vi "CRYUnflatten SoundCard.vi"(11 "Flatten SoundCard":string) -> (0 "Error?":bool=TRUE, 2 "SoundCard":T1={"Name"="", "Analog I/O"=0, "Digital I/O"=0, "Channels"=2, "Dig Dev ID"=1, "N ports"=3, "Interface"=0, "Dig I/O Ports"=[{"port #"=1, "width"=8, "direction"=0}, {"port #"=2, "width"=8, "direction"=0}, {"port #"=3, "width"=8, "direction"=0}], "Interf settings"=[], "N interfs"=3, "udev SNs"=[], "udev enable"=FALSE, "Channel Array"=[], "Cal sequence"="", "SelectedIn"=0, "SelectedOut"=0, "SelectedTab"=0, "State"=FALSE, "Help"="", "Advanced"=FALSE, "In Audio Driver"=0, "Out Audio Driver"=0} {"Channel Array"."Coupling" items=["Default"=-1, "RSE"=10083, "NRSE"=10078, "Differential"=10106, "Pseudodifferential"=12529]; "Channel Array"."term config" items=["Default"=-1, "RSE"=10083, "NRSE"=10078, "Differential"=10106, "Pseudodifferential"=12529]; "Channel Array"."Anti-aliasing Factor (%fs)" format="%.2f"}, 3 "Header info":T3={"Data type"="Data            ", "Version"=1, "Dimensions"=0})   [LabVIEW 2013]
uses:
  Typedef Control/CRYHardware.ctl
  Typedef Control/CRYHardware Channel Info.ctl
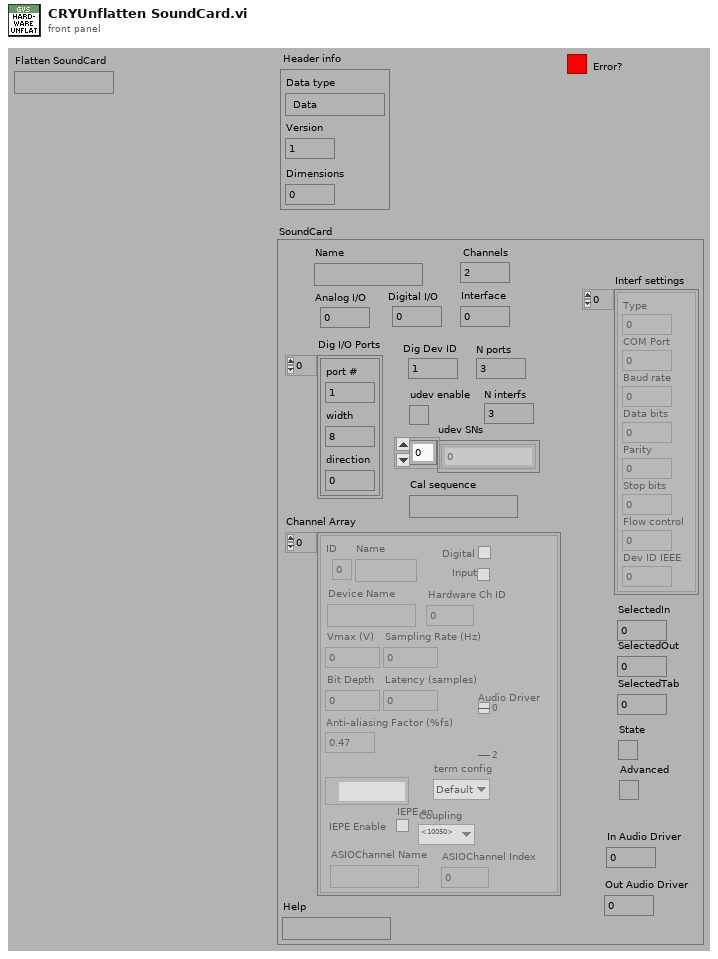
[diagram p1: front panel]
types:
  T1 = typedef "CRYHardware.ctl" = cluster{"Name":string, "Analog I/O":u16, "Digital I/O":u16, "Channels":u8, "Dig Dev ID":u8, "N ports":u8, "Interface":u32, "Dig I/O Ports":cluster{"port #":i16, "width":i16, "direction":i32}[], "Interf settings":cluster{"Type":u16, "COM Port":u8, "Baud rate":u32, "Data bits":u32, "Parity":u16, "Stop bits":u16, "Flow control":u16, "Dev ID IEEE":u8}[], "N interfs":i32, "udev SNs":i16[], "udev enable":bool, "Channel Array":T2[], "Cal sequence":string, "SelectedIn":u16, "SelectedOut":u16, "SelectedTab":u16, "State":bool, "Help":string, "Advanced":bool, "In Audio Driver":u16, "Out Audio Driver":u16}
  T2 = typedef "CRYHardware Channel Info.ctl" = cluster{"ID":i32, "Name":string, "Digital":bool, "Input":bool, "Device Name":string, "Hardware Ch ID":u8, "Vmax (V)":dbl, "Latency (samples)":dbl, "Sampling Rate (Hz)":u32, "Bit Depth":u32, "Anti-aliasing Factor (%fs)":sgl, "DAQmx Channel":tag, "term config":i32, "Coupling":i32, "IEPE en":bool, "ASIOChannel Name":string, "Audio Driver":u16, "ASIOChannel Index":u8}
  T3 = cluster{"Data type":string, "Version":u16, "Dimensions":u8}
  T4 = cluster{"Name":string, "Analog I/O":u16, "Digital I/O":u16, "Channels":u8, "Dig Dev ID":u8, "N ports":u8, "Interface":u32, "Dig I/O Ports":cluster{"port #":i16, "width":i16, "direction":i32}[], "Interf settings":cluster{"Type":u16, "COM Port":u8, "Baud rate":u32, "Data bits":u32, "Parity":u16, "Stop bits":u16, "Flow control":u16, "Dev ID IEEE":u8}[], "N interfs":i32, "udev SNs":i16[], "udev enable":bool, "Channel Array":cluster{"ID":i32, "Name":string, "Digital":bool, "Input":bool, "Device Name":string, "Hardware Ch ID":u8, "Vmax (V)":dbl, "Latency (samples)":dbl, "Sampling Rate (Hz)":u32, "Bit Depth":u32, "Anti-aliasing Factor (%fs)":sgl, "DAQmx Channel":tag, "term config":i32, "Coupling":i32, "IEPE en":bool, "Audio Driver":u16}[], "Cal sequence":string, "SelectedIn":u16, "SelectedOut":u16, "SelectedTab":u16, "State":bool, "Help":string, "Advanced":bool}
  T5 = cluster{"Name":string, "Analog I/O":u16, "Digital I/O":u16, "Channels":u8, "Dig Dev ID":u8, "N ports":u8, "Interface":u32, "Dig I/O Ports":cluster{"port #":i16, "width":i16, "direction":i32}[], "Interf settings":cluster{"Type":u16, "COM Port":u8, "Baud rate":u32, "Data bits":u32, "Parity":u16, "Stop bits":u16, "Flow control":u16, "Dev ID IEEE":u8}[], "N interfs":i32, "udev SNs":i16[], "udev enable":bool, "Channel Array":cluster{"ID":i32, "Name":string, "Digital":bool, "Input":bool, "Device Name":string, "Hardware Ch ID":u8, "Vmax (V)":dbl, "Latency (samples)":dbl, "Sampling Rate (Hz)":u32, "Bit Depth":u32, "Anti-aliasing Factor (%fs)":sgl, "DAQmx Channel":tag, "term config":i32, "Coupling":i32, "IEPE en":bool, "Audio Driver":u16}[], "Cal sequence":string, "SelectedIn":u16, "SelectedOut":u16, "SelectedTab":u16, "State":bool, "Help":string}
  T6 = cluster{"Name":string, "Analog I/O":u16, "Digital I/O":u16, "Channels":u8, "Dig Dev ID":u8, "N ports":u8, "Interface":u32, "Dig I/O Ports":cluster{"port #":i16, "width":i16, "direction":i32}[], "Interf settings":cluster{"Type":u16, "COM Port":u8, "Baud rate":u32, "Data bits":u32, "Parity":u16, "Stop bits":u16, "Flow control":u16, "Dev ID IEEE":u8}[], "N interfs":i32, "udev SNs":i16[], "udev enable":bool, "Channel Array":cluster{"ID":i32, "Name":string, "Digital":bool, "Input":bool, "Device Name":string, "Hardware Ch ID":u8, "Vmax (V)":dbl, "Latency (samples)":dbl, "Sampling Rate (Hz)":u32, "Bit Depth":u32, "Anti-aliasing Factor (%fs)":sgl, "DAQmx Channel":tag, "term config":i32, "Coupling":i32, "IEPE en":bool, "Audio Driver":u16}[], "Cal sequence":string, "SelectedIn":u16, "SelectedOut":u16, "SelectedTab":u16, "State":bool}
  T7 = cluster{"unsigned byte array[0]":u8, "unsigned byte array[1]":u8, "unsigned byte array[2]":u8}
  T8 = cluster{"port #":i16, "width":i16, "direction":i32}[]
  T9 = cluster{"Type":u16, "COM Port":u8, "Baud rate":u32, "Data bits":u32, "Parity":u16, "Stop bits":u16, "Flow control":u16, "Dev ID IEEE":u8}[]
  T10 = cluster{"ID":i32, "Name":string, "Digital":bool, "Input":bool, "Device Name":string, "Hardware Ch ID":u8, "Vmax (V)":dbl, "Latency (samples)":dbl, "Sampling Rate (Hz)":u32, "Bit Depth":u32, "Anti-aliasing Factor (%fs)":sgl, "DAQmx Channel":tag, "term config":i32, "Coupling":i32, "IEPE en":bool, "Audio Driver":u16}[]
  T11 = cluster{"substring":string, u16, "unsigned byte array[2]":u8}
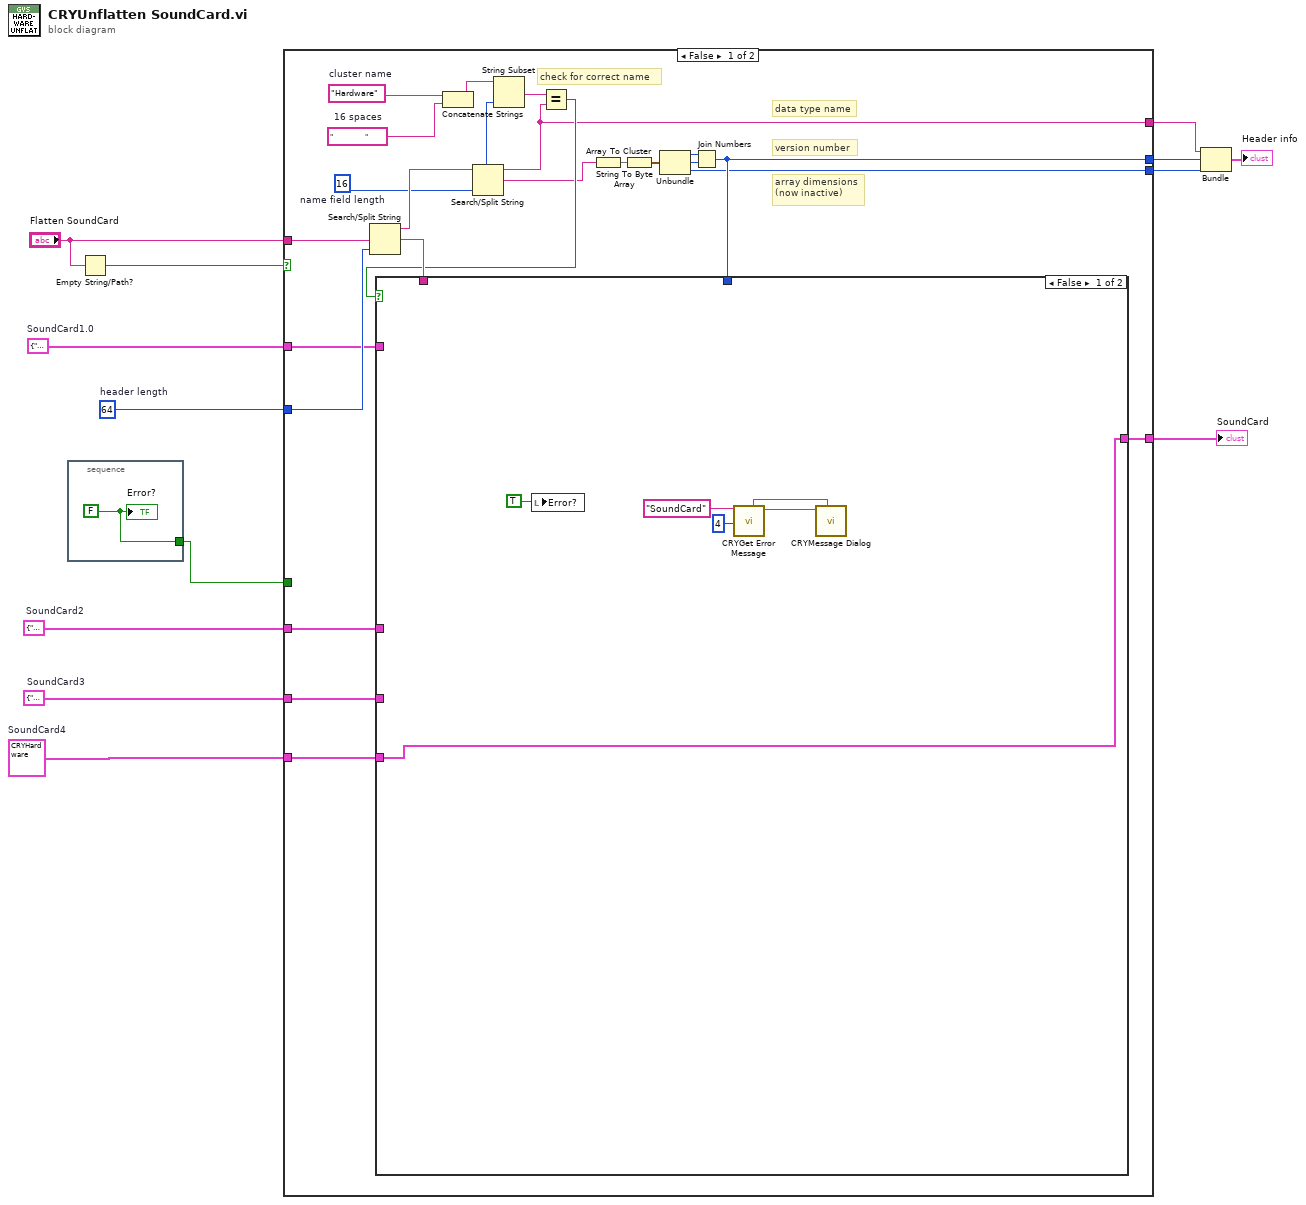
[diagram p0: block diagram]
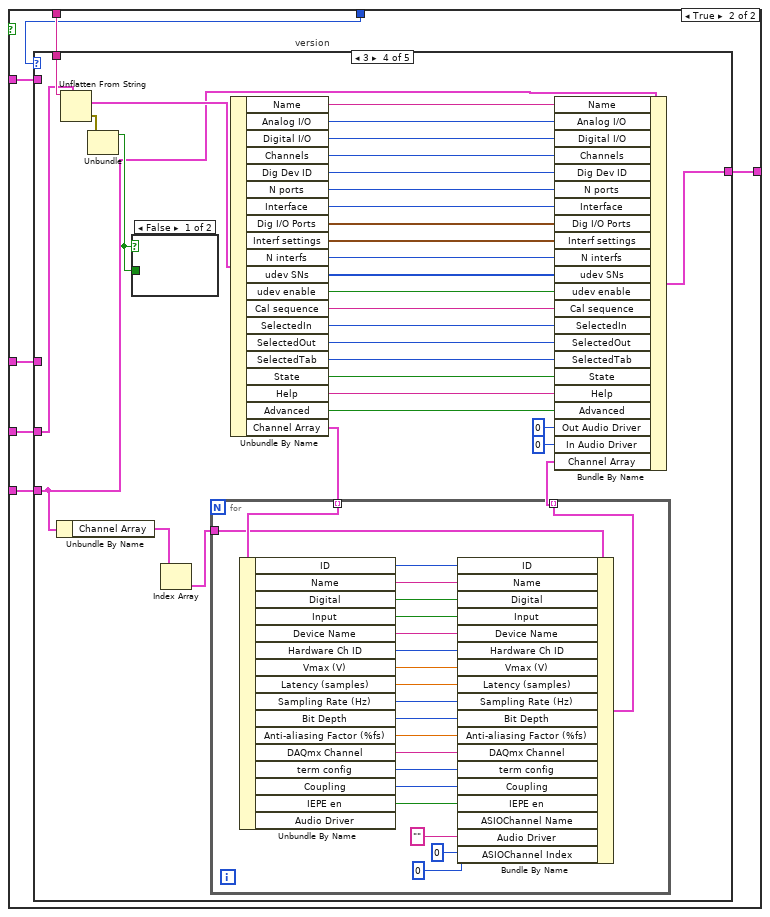
[diagram p2: hidden frame]
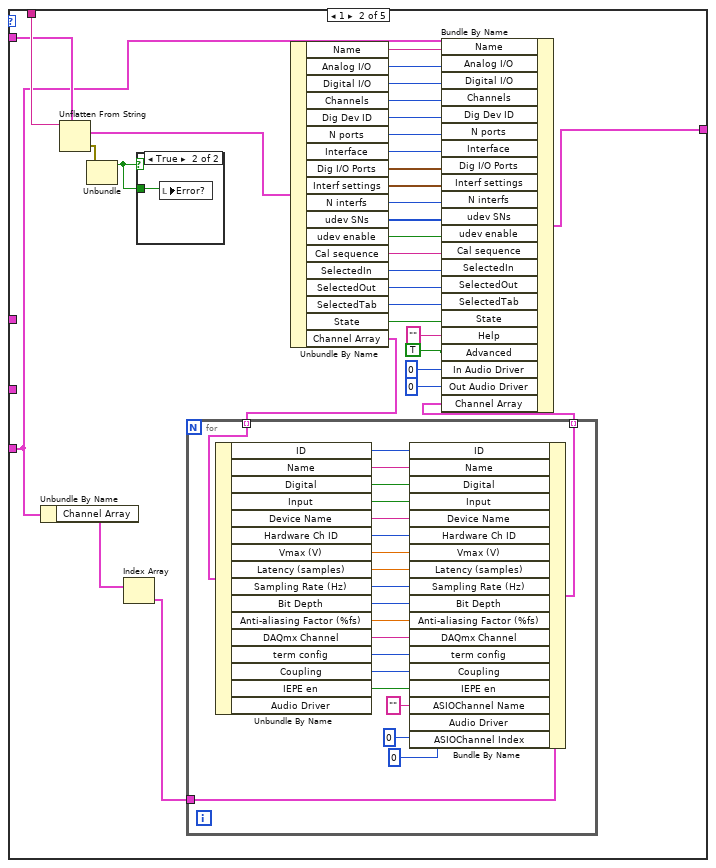
[diagram p4: hidden frame]
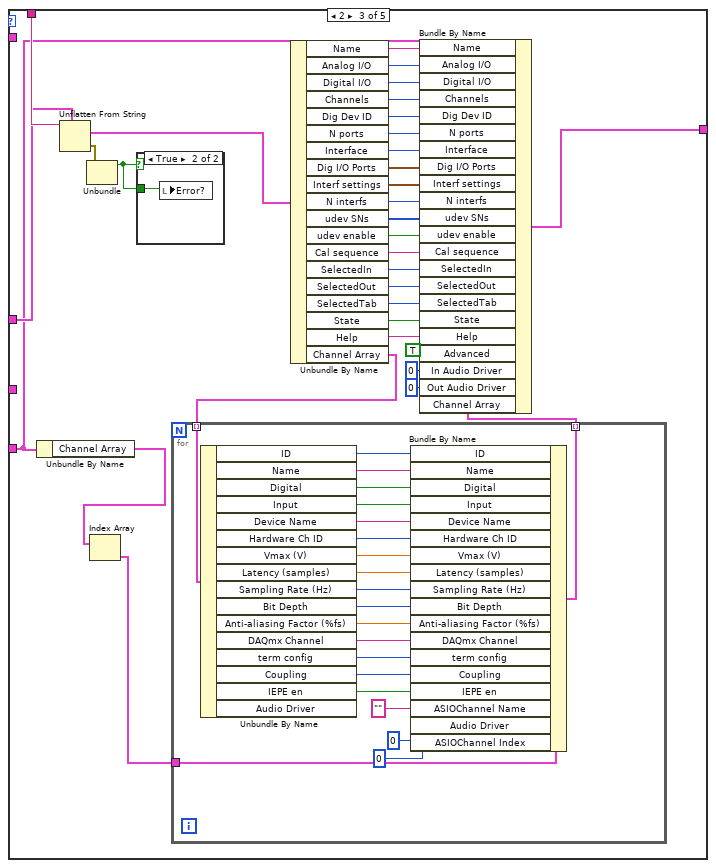
[diagram p6: hidden frame]
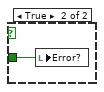
[diagram p8: hidden frame]
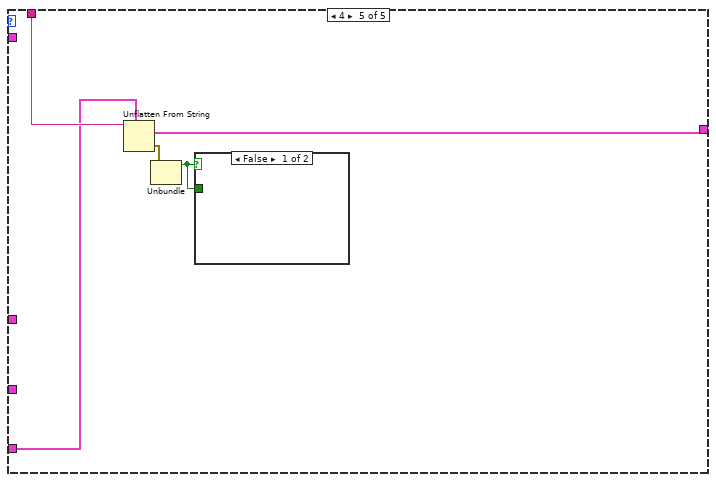
[diagram p9: hidden frame]
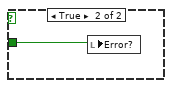
[diagram p10: hidden frame]
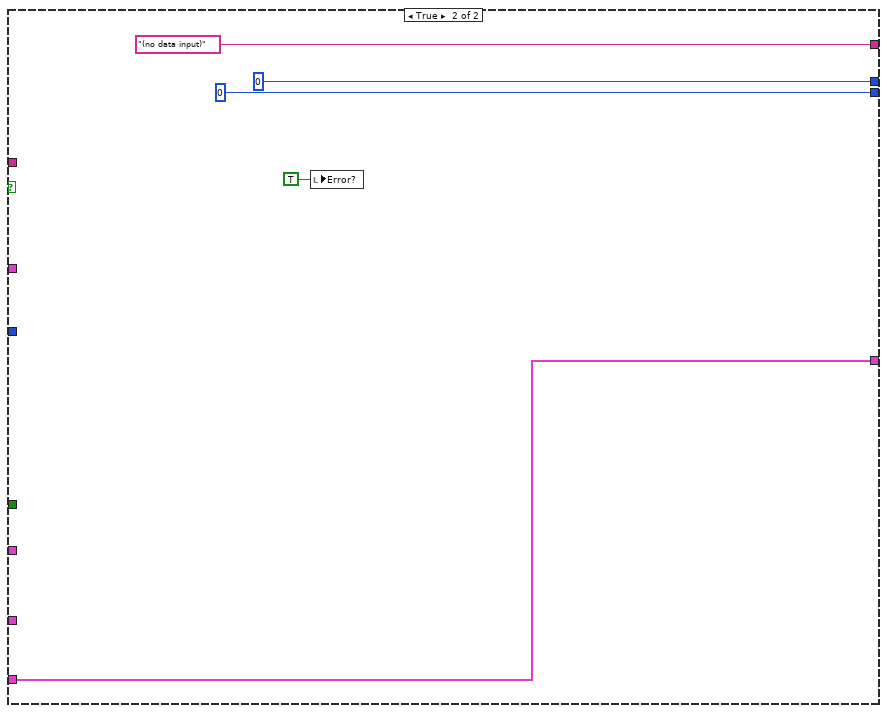
[diagram p11: hidden frame]
diagram:
  w1 = T1 {"Name"="CardDeluxe Analog", "Analog I/O"=0, "Digital I/O"=0, "Channels"=2, "Dig Dev ID"=1, "N ports"=3, "Interface"=0, "Dig I/O Ports"=[{"port #"=1, "width"=8, "direction"=0}, {"port #"=2, "width"=8, "direction"=0}, {"port #"=3, "width"=8, "direction"=0}], "Interf settings"=[], "N interfs"=3, "udev SNs"=[], "udev enable"=FALSE, "Channel Array"=[], "Cal sequence"="", "SelectedIn"=0, "SelectedOut"=0, "SelectedTab"=0, "State"=FALSE, "Help"="", "Advanced"=TRUE, "In Audio Driver"=0, "Out Audio Driver"=0}  # SoundCard4
  w2 = T4 {"Name"="CardDeluxe Analog", "Analog I/O"=0, "Digital I/O"=0, "Channels"=2, "Dig Dev ID"=1, "N ports"=3, "Interface"=0, "Dig I/O Ports"=[{"port #"=1, "width"=8, "direction"=0}, {"port #"=2, "width"=8, "direction"=0}, {"port #"=3, "width"=8, "direction"=0}], "Interf settings"=[], "N interfs"=3, "udev SNs"=[], "udev enable"=FALSE, "Channel Array"=[], "Cal sequence"="", "SelectedIn"=0, "SelectedOut"=0, "SelectedTab"=0, "State"=FALSE, "Help"="", "Advanced"=TRUE}  # SoundCard3
  w3 = T5 {"Name"="", "Analog I/O"=0, "Digital I/O"=0, "Channels"=2, "Dig Dev ID"=1, "N ports"=3, "Interface"=0, "Dig I/O Ports"=[{"port #"=0, "width"=0, "direction"=0}, {"port #"=2, "width"=8, "direction"=0}, {"port #"=3, "width"=8, "direction"=0}], "Interf settings"=[], "N interfs"=3, "udev SNs"=[], "udev enable"=FALSE, "Channel Array"=[], "Cal sequence"="", "SelectedIn"=0, "SelectedOut"=0, "SelectedTab"=0, "State"=FALSE, "Help"=""}  # SoundCard2
  w4 = T6 {"Name"="", "Analog I/O"=0, "Digital I/O"=0, "Channels"=2, "Dig Dev ID"=1, "N ports"=3, "Interface"=0, "Dig I/O Ports"=[{"port #"=0, "width"=0, "direction"=0}, {"port #"=2, "width"=8, "direction"=0}, {"port #"=3, "width"=8, "direction"=0}], "Interf settings"=[], "N interfs"=3, "udev SNs"=[], "udev enable"=FALSE, "Channel Array"=[], "Cal sequence"="", "SelectedIn"=0, "SelectedOut"=0, "SelectedTab"=0, "State"=FALSE}  # SoundCard1.0
  w11 = 64  # header length
  n1 = stacked-sequence {
    tunnel: [w14] -> w6
    frame #0 {
      w14 = FALSE
      "Error?" <- w14
    }
  }
  n2 = Empty String/Path?(string/path="Flatten SoundCard") -> (empty?=w12:bool)
  n3 = case shown="False" w12 {
    tunnel: "Flatten SoundCard" -> [w37 _]
    tunnel: w11 -> [w31 _]
    tunnel: [w28 u16 0] -> w9
    tunnel: [w20 u8 0] -> w10
    tunnel: [w21 "(no data input)" ("substring")] -> w8
    tunnel: w6 -> [_ _]
    tunnel: [w19 w220] -> w5
    tunnel: w4 -> [w18 _]
    tunnel: w3 -> [w17 _]
    tunnel: w2 -> [w16 _]
    tunnel: w1 -> [w15 w220]
    frame False {
      w25 = "                "  # 16 spaces
      w26 = "Hardware"  # cluster name
      w23 = 16  # name field length
      # "check for correct name"
      # "array dimensions\n(now inactive)"
      # "version number"
      # "data type name"
      n4 = Search/Split String(string=w37, offset (0)=w31) -> (substring before match=w30:string, match + rest of string=w32:string)  [unwired: 2 out]
      n5 = Concatenate Strings(w26, w25) -> (w24:string)
      n6 = Search/Split String(string=w30, offset (0)=w23) -> (substring before match=w21:string, match + rest of string=w27:string)  [unwired: 2 out]
      n7 = String Subset(string=w24, length (rest)=w23) -> (substring=w22:string)  [unwired: 1 out]
      n8 = Equal?(x=w22, y=w21) -> (x = y?=w29:bool)
      n9 = String To Byte Array(string=w27) -> (unsigned byte array=w36:u8[])
      n10 = Array To Cluster(array=w36) -> (cluster=w35:T7)
      n11 = Unbundle(w35) -> ("unsigned byte array[0]"=w34:u8, "unsigned byte array[1]"=w33:u8, "unsigned byte array[2]"=w20:u8)
      n12 = Join Numbers(hi=w34, lo=w33) -> ((hi.lo)=w28:u16)
      n13 = case shown="False" w29 {
        tunnel: w32 -> [_ w50]
        tunnel: w28 -> [_ w49]
        tunnel: [w38 w48] -> w19
        tunnel: w18 -> [_ w47]
        tunnel: w17 -> [_ w46]
        tunnel: w16 -> [_ w45]
        tunnel: w15 -> [w38 w44]
        frame False {
          n14 = local write "Error?"(TRUE) -> ()
          n15 = call "CRYGet Error Message.vi"("Error No"=4 ("No"), "Kind"="SoundCard") -> ("Message"=w40:string, "Window Title"=w39:string)  [unwired: 4 in, 4 out]
          n16 = call "CRYMessage Dialog.vi"("Window Title"=w39, "Message Content"=w40) -> ()  [unwired: 8 in, 2 out]
        }
        frame True {
          n17 = case "version" shown="3" w49 {
            tunnel: w50 -> [_ w83 w137 w191 w218]
            tunnel: [w51 w78 w133 w164 w215] -> w48
            tunnel: w47 -> [_ w80 _ _ _]
            tunnel: w46 -> [_ _ w114 _ _]
            tunnel: w45 -> [_ _ _ w188 _]
            tunnel: w44 -> [w51 w58 w110 w166 w214]
            frame Default {
            }
            frame 1 {
              n18 = Unbundle By Name(w58) -> ("Channel Array"=w53:T2[])
              n19 = Unflatten From String(type=w80, binary string=w83) -> (value=w79:T6, error out=w81:errorcluster)  [unwired: 1 in, 3 out]
              n20 = Unbundle(w81) -> ("status"=w82:bool)  [unwired: 2 out]
              n21 = Index Array(array=w53) -> (element=w52:T2)  [unwired: 1 in]
              n22 = case shown="True" w82 {
                tunnel: w82 -> [_ w105]
                frame False {
                }
                frame True {
                  n23 = local write "Error?"(w105) -> ()
                }
              }
              n24 = Unbundle By Name(w79) -> ("Name"=w77:string, "Analog I/O"=w76:u16, "Digital I/O"=w75:u16, "Channels"=w74:u8, "Dig Dev ID"=w73:u8, "N ports"=w72:u8, "Interface"=w71:u32, "Dig I/O Ports"=w70:T8, "Interf settings"=w69:T9, "N interfs"=w68:i32, "udev SNs"=w67:i16[], "udev enable"=w66:bool, "Cal sequence"=w65:string, "SelectedIn"=w64:u16, "SelectedOut"=w63:u16, "SelectedTab"=w62:u16, "State"=w61:bool, "Channel Array"=w57:T10)
              n25 = for {
                tunnel: w52 -> [w104]
                tunnel: [w86] -> w56 mode=indexing
                tunnel: w57 -> [w85] mode=indexing
                n26 = Unbundle By Name(w85) -> ("ID"=w103:i32, "Name"=w102:string, "Digital"=w101:bool, "Input"=w100:bool, "Device Name"=w99:string, "Hardware Ch ID"=w98:u8, "Vmax (V)"=w97:dbl, "Latency (samples)"=w96:dbl, "Sampling Rate (Hz)"=w95:u32, "Bit Depth"=w94:u32, "Anti-aliasing Factor (%fs)"=w93:sgl, "DAQmx Channel"=w92:tag, "term config"=w91:i32, "Coupling"=w90:i32, "IEPE en"=w89:bool)  [unwired: 1 out]
                n27 = Bundle By Name(cluster=w104, "ID"=w103, "Name"=w102, "Digital"=w101, "Input"=w100, "Device Name"=w99, "Hardware Ch ID"=w98, "Vmax (V)"=w97, "Latency (samples)"=w96, "Sampling Rate (Hz)"=w95, "Bit Depth"=w94, "Anti-aliasing Factor (%fs)"=w93, "DAQmx Channel"=w92, "term config"=w91, "Coupling"=w90, "IEPE en"=w89, "ASIOChannel Name"="", "Audio Driver"=u16 0, "ASIOChannel Index"=u8 0) -> (w86:T2)
              }
              n28 = Bundle By Name(cluster=w58, "Name"=w77, "Analog I/O"=w76, "Digital I/O"=w75, "Channels"=w74, "Dig Dev ID"=w73, "N ports"=w72, "Interface"=w71, "Dig I/O Ports"=w70, "Interf settings"=w69, "N interfs"=w68, "udev SNs"=w67, "udev enable"=w66, "Cal sequence"=w65, "SelectedIn"=w64, "SelectedOut"=w63, "SelectedTab"=w62, "State"=w61, "Help"="", "Advanced"=TRUE, "In Audio Driver"=u16 0 ("Audio Driver"), "Out Audio Driver"=u16 0, "Channel Array"=w56) -> (w78:T1)
            }
            frame 2 {
              n29 = Unbundle By Name(w110) -> ("Channel Array"=w107:T2[])
              n30 = Unflatten From String(type=w114, binary string=w137) -> (value=w134:T5, error out=w135:errorcluster)  [unwired: 1 in, 3 out]
              n31 = Unbundle(w135) -> ("status"=w136:bool)  [unwired: 2 out]
              n32 = Index Array(array=w107) -> (element=w106:T2)  [unwired: 1 in]
              n33 = case shown="True" w136 {
                tunnel: w136 -> [_ w159]
                frame False {
                }
                frame True {
                  n34 = local write "Error?"(w159) -> ()
                }
              }
              n35 = Unbundle By Name(w134) -> ("Name"=w132:string, "Analog I/O"=w131:u16, "Digital I/O"=w130:u16, "Channels"=w129:u8, "Dig Dev ID"=w128:u8, "N ports"=w127:u8, "Interface"=w126:u32, "Dig I/O Ports"=w125:T8, "Interf settings"=w124:T9, "N interfs"=w123:i32, "udev SNs"=w122:i16[], "udev enable"=w121:bool, "Cal sequence"=w120:string, "SelectedIn"=w119:u16, "SelectedOut"=w118:u16, "SelectedTab"=w117:u16, "State"=w116:bool, "Help"=w113:string, "Channel Array"=w112:T10)
              n36 = for {
                tunnel: w112 -> [w158] mode=indexing
                tunnel: w106 -> [w157]
                tunnel: [w139] -> w111 mode=indexing
                n37 = Unbundle By Name(w158) -> ("ID"=w156:i32, "Name"=w155:string, "Digital"=w154:bool, "Input"=w153:bool, "Device Name"=w152:string, "Hardware Ch ID"=w151:u8, "Vmax (V)"=w150:dbl, "Latency (samples)"=w149:dbl, "Sampling Rate (Hz)"=w148:u32, "Bit Depth"=w147:u32, "Anti-aliasing Factor (%fs)"=w146:sgl, "DAQmx Channel"=w145:tag, "term config"=w144:i32, "Coupling"=w143:i32, "IEPE en"=w142:bool)  [unwired: 1 out]
                n38 = Bundle By Name(cluster=w157, "ID"=w156, "Name"=w155, "Digital"=w154, "Input"=w153, "Device Name"=w152, "Hardware Ch ID"=w151, "Vmax (V)"=w150, "Latency (samples)"=w149, "Sampling Rate (Hz)"=w148, "Bit Depth"=w147, "Anti-aliasing Factor (%fs)"=w146, "DAQmx Channel"=w145, "term config"=w144, "Coupling"=w143, "IEPE en"=w142, "ASIOChannel Name"="", "Audio Driver"=u16 0, "ASIOChannel Index"=u8 0) -> (w139:T2)
              }
              n39 = Bundle By Name(cluster=w110, "Name"=w132, "Analog I/O"=w131, "Digital I/O"=w130, "Channels"=w129, "Dig Dev ID"=w128, "N ports"=w127, "Interface"=w126, "Dig I/O Ports"=w125, "Interf settings"=w124, "N interfs"=w123, "udev SNs"=w122, "udev enable"=w121, "Cal sequence"=w120, "SelectedIn"=w119, "SelectedOut"=w118, "SelectedTab"=w117, "State"=w116, "Help"=w113, "Advanced"=TRUE, "In Audio Driver"=u16 0 ("Audio Driver"), "Out Audio Driver"=u16 0 ("In Audio Driver"), "Channel Array"=w111) -> (w133:T1)
            }
            frame 3 {
              n40 = Unbundle By Name(w166) -> ("Channel Array"=w161:T2[])
              n41 = Unflatten From String(type=w188, binary string=w191) -> (value=w187:T4, error out=w189:errorcluster)  [unwired: 1 in, 3 out]
              n42 = Unbundle(w189) -> ("status"=w190:bool)  [unwired: 2 out]
              n43 = case shown="False" w190 {
                tunnel: w190 -> [_ w213]
                frame False {
                }
                frame True {
                  n44 = local write "Error?"(w213) -> ()
                }
              }
              n45 = Index Array(array=w161) -> (element=w160:T2)  [unwired: 1 in]
              n46 = Unbundle By Name(w187) -> ("Name"=w186:string, "Analog I/O"=w185:u16, "Digital I/O"=w184:u16, "Channels"=w183:u8, "Dig Dev ID"=w182:u8, "N ports"=w181:u8, "Interface"=w180:u32, "Dig I/O Ports"=w179:T8, "Interf settings"=w178:T9, "N interfs"=w177:i32, "udev SNs"=w176:i16[], "udev enable"=w175:bool, "Cal sequence"=w174:string, "SelectedIn"=w173:u16, "SelectedOut"=w172:u16, "SelectedTab"=w171:u16, "State"=w170:bool, "Help"=w169:string, "Advanced"=w168:bool, "Channel Array"=w167:T10)
              n47 = for {
                tunnel: w167 -> [w212] mode=indexing
                tunnel: w160 -> [w194]
                tunnel: [w193] -> w165 mode=indexing
                n48 = Unbundle By Name(w212) -> ("ID"=w211:i32, "Name"=w210:string, "Digital"=w209:bool, "Input"=w208:bool, "Device Name"=w207:string, "Hardware Ch ID"=w206:u8, "Vmax (V)"=w205:dbl, "Latency (samples)"=w204:dbl, "Sampling Rate (Hz)"=w203:u32, "Bit Depth"=w202:u32, "Anti-aliasing Factor (%fs)"=w201:sgl, "DAQmx Channel"=w200:tag, "term config"=w199:i32, "Coupling"=w198:i32, "IEPE en"=w197:bool)  [unwired: 1 out]
                n49 = Bundle By Name(cluster=w194, "ID"=w211, "Name"=w210, "Digital"=w209, "Input"=w208, "Device Name"=w207, "Hardware Ch ID"=w206, "Vmax (V)"=w205, "Latency (samples)"=w204, "Sampling Rate (Hz)"=w203, "Bit Depth"=w202, "Anti-aliasing Factor (%fs)"=w201, "DAQmx Channel"=w200, "term config"=w199, "Coupling"=w198, "IEPE en"=w197, "ASIOChannel Name"="", "Audio Driver"=u16 0, "ASIOChannel Index"=u8 0) -> (w193:T2)
              }
              n50 = Bundle By Name(cluster=w166, "Name"=w186, "Analog I/O"=w185, "Digital I/O"=w184, "Channels"=w183, "Dig Dev ID"=w182, "N ports"=w181, "Interface"=w180, "Dig I/O Ports"=w179, "Interf settings"=w178, "N interfs"=w177, "udev SNs"=w176, "udev enable"=w175, "Cal sequence"=w174, "SelectedIn"=w173, "SelectedOut"=w172, "SelectedTab"=w171, "State"=w170, "Help"=w169, "Advanced"=w168, "Out Audio Driver"=u16 0 ("Audio Driver"), "In Audio Driver"=u16 0, "Channel Array"=w165) -> (w164:T1)
            }
            frame 4 {
              n51 = Unflatten From String(type=w214, binary string=w218) -> (value=w215:T1, error out=w216:errorcluster)  [unwired: 1 in, 3 out]
              n52 = Unbundle(w216) -> ("status"=w217:bool)  [unwired: 2 out]
              n53 = case shown="False" w217 {
                tunnel: w217 -> [_ w219]
                frame False {
                }
                frame True {
                  n54 = local write "Error?"(w219) -> ()
                }
              }
            }
          }
        }
      }
    }
    frame True {
      n55 = local write "Error?"(TRUE ("Error?")) -> ()
    }
  }
  "SoundCard" <- w5
  n56 = Bundle("substring"=w8, w9, "unsigned byte array[2]"=w10) -> (→"Header info":T11)  [unwired: 1 out]
